vi "Purge_PDop_00.vi"() -> ()   [LabVIEW 2011]
panel:
  in  "stop":bool
  in  "tot fill wait":dbl=300.0 caption="total fill wait (s)"
  in  "tot evac wait":dbl=300.0 caption="total evacuation wait (s)"
  out "Numeric":i32 caption="iteration"
  in  "Iterations":i32=20
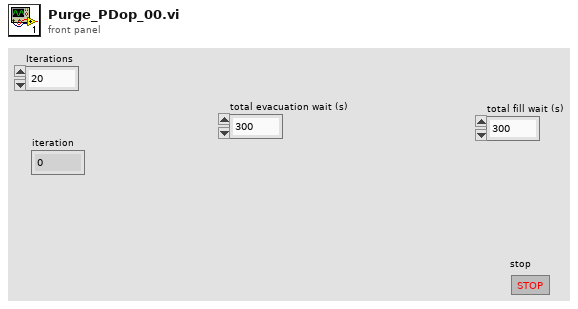
[diagram p1: front panel]
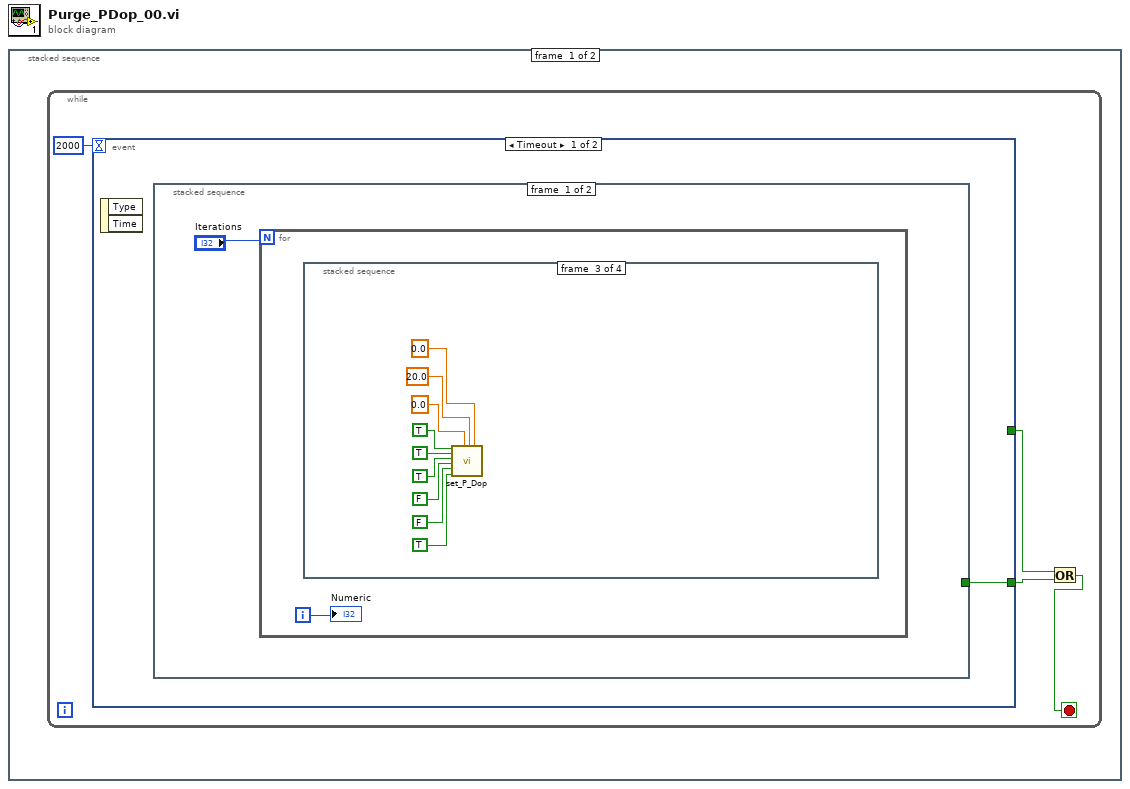
[diagram p0: block diagram]
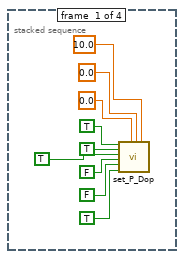
[diagram p2: hidden frame]
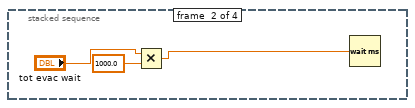
[diagram p3: hidden frame]
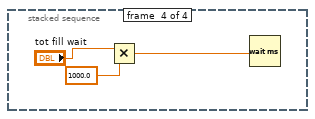
[diagram p4: hidden frame]
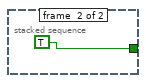
[diagram p5: hidden frame]
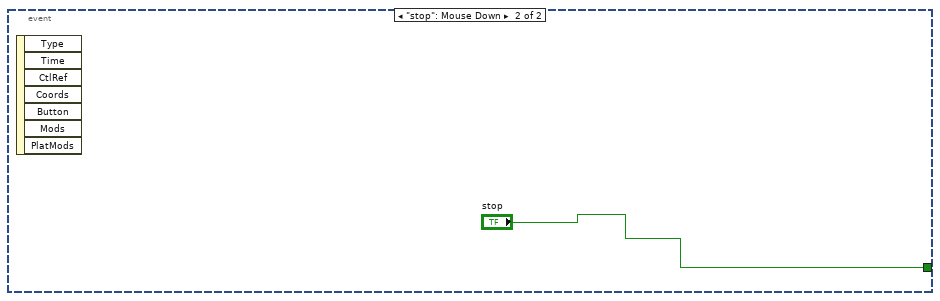
[diagram p6: hidden frame]
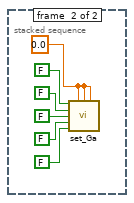
[diagram p7: hidden frame]
diagram:
  n1 = stacked-sequence {
    frame #0 {
      n2 = while {
        stop <- w2 stop-if-true
        n3 = event shown="[0] Timeout" {
          selector: _ -> [_ _]
          dyn-events: _ -> [_ _]
          timeout: 2000 -> [_ _]
          tunnel: [_ "stop"] -> w3
          tunnel: [w5 _] -> w4
          event Timeout {
            n4 = event-data() -> ()  [unwired: 1 in, 2 out]
            n5 = stacked-sequence {
              tunnel: [_ TRUE] -> w5
              frame #0 {
                n6 = for {
                  N: "Iterations" -> [_]
                  i -> [w7]
                  n7 = stacked-sequence {
                    frame #0 {
                      n8 = call "set_P_Dop.vi"("P_Dop Active"=TRUE ("As_Gas Active"), "P_Dop Bubbler"=TRUE ("As_Gas In"), "P_Dop H2 Dilute"=TRUE, "P_Dop Gas Source"=FALSE ("As_Gas H2"), "P_Dop Run"=FALSE ("As_Gas Run"), "P_Dop Remote"=TRUE ("As_Gas Remote"), "P_Dop Flow 3"=0.0 ("As_Gas Flow"), "P_Dop Flow 2"=0.0 ("Ga Flow 2"), "P_Dop Flow 1"=10.0 ("Ga Flow 1")) -> ()  [unwired: 11 in]
                    }
                    frame #1 {
                      n9 = Multiply(x="tot evac wait", y=1000.0) -> (x*y=w17:dbl)
                      n10 = Wait (ms)(milliseconds to wait=w17) -> ()  [unwired: 1 out]
                    }
                    frame #2 {
                      n11 = call "set_P_Dop.vi"("P_Dop Active"=TRUE ("As_Gas Active"), "P_Dop Bubbler"=TRUE ("As_Gas In"), "P_Dop H2 Dilute"=TRUE, "P_Dop Gas Source"=FALSE ("As_Gas H2"), "P_Dop Run"=FALSE ("As_Gas Run"), "P_Dop Remote"=TRUE ("As_Gas Remote"), "P_Dop Flow 3"=0.0, "P_Dop Flow 2"=20.0 ("Ga Flow 2"), "P_Dop Flow 1"=0.0 ("As_Gas Flow")) -> ()  [unwired: 11 in]
                    }
                    frame #3 {
                      n12 = Multiply(x="tot fill wait", y=1000.0) -> (x*y=w29:dbl)
                      n13 = Wait (ms)(milliseconds to wait=w29) -> ()  [unwired: 1 out]
                    }
                  }
                  "Numeric" <- w7
                }
              }
              frame #1 {
              }
            }
          }
          event "stop": Mouse Down {
            n14 = event-data() -> ()  [unwired: 1 in, 7 out]
          }
        }
        n15 = Or(x=w3, y=w4) -> (x .or. y?=w2:bool)
      }
    }
    frame #1 {
      w34 = 0.0 ("As_Gas Flow")
      n16 = call "set_Ga.vi"("Ga Active"=FALSE ("As_Gas Active"), "Ga Flow 3"=w34, "Ga Flow 2"=w34, "Ga Flow 1"=w34, "Ga Bubbler"=FALSE ("As_Gas In"), "Ga H2 Dilute"=FALSE ("As_Gas H2"), "Ga Run"=FALSE ("As_Gas Run"), "Ga Remote"=FALSE ("As_Gas Remote")) -> ()  [unwired: 8 in]
    }
  }
